vi "Filter.vi"(4 "Lower Cut-Off 2":dbl=15000.0 caption="Lower Cut-Off", 5 "Upper Cut-Off 2":dbl=400.0 caption="Upper Cut-Off", 6 "Lower Cut-Off":dbl=15000.0, 7 "Upper Cut-Off":dbl=400.0, 8 "Input Waveform 2":waveform(dbl), 11 "Input Waveform":waveform(dbl)) -> (0 "Filtered Signal 2":dynamicdata(graph) caption="Filtered Signal", 3 "Filtered Signal":dynamicdata(graph))   [LabVIEW 2014]
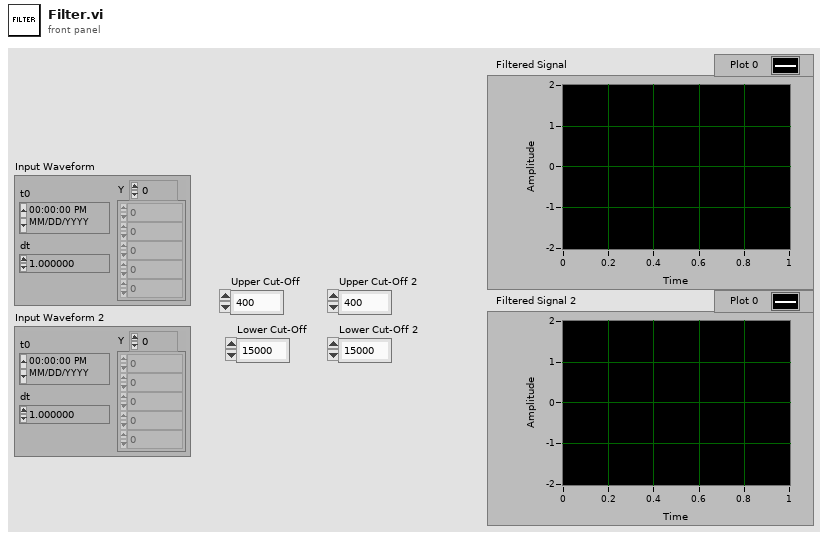
[diagram p1: front panel]
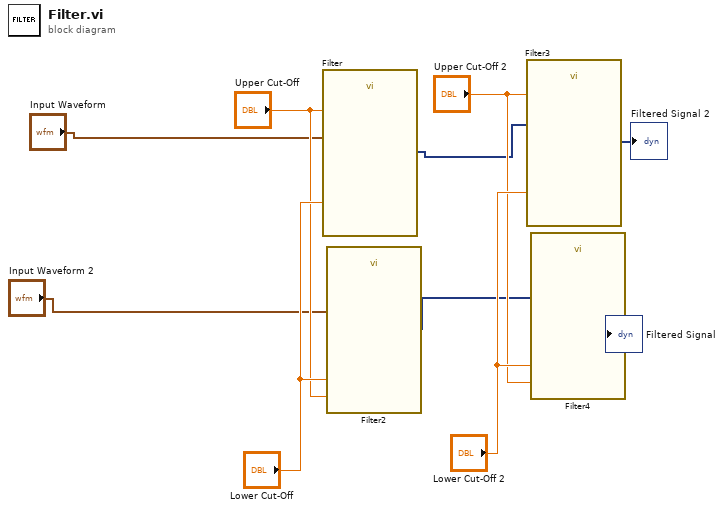
[diagram p0: block diagram]
diagram:
  n1 = call "Filter"("Lower Cut-Off"="Lower Cut-Off", "Upper Cut-Off"="Upper Cut-Off", "Signal"="Input Waveform") -> ("Filtered Signal"=w6:dynamicdata)  [unwired: 7 in, 1 out]
  n2 = call "Filter2"("Lower Cut-Off"="Lower Cut-Off", "Upper Cut-Off"="Upper Cut-Off", "Signal"="Input Waveform 2") -> ("Filtered Signal"=w5:dynamicdata)  [unwired: 7 in, 1 out]
  n3 = call "Filter3"("Lower Cut-Off"="Lower Cut-Off 2", "Upper Cut-Off"="Upper Cut-Off 2", "Signal"=w6) -> ("Filtered Signal"=→"Filtered Signal 2":dynamicdata)  [unwired: 7 in, 1 out]
  n4 = call "Filter4"("Lower Cut-Off"="Lower Cut-Off 2", "Upper Cut-Off"="Upper Cut-Off 2", "Signal"=w5) -> ("Filtered Signal"=→"Filtered Signal":dynamicdata)  [unwired: 7 in, 1 out]
